vi "TCP Factory.vi"(8 "error in (no error)":errorcluster, 10 "TCP Settings":cluster{"IP Address":string, "Port":u16}) -> (0 "error out":errorcluster, 3 "TCP out":refnum<class "TCP.lvclass">)   [LabVIEW 2019, in "Protocols.lvlib" / "TCP.lvclass"]
uses:
  TCP.lvclass
  TCP.lvclass/TCP.ctl
  Data Access/Write IP Address.vi
  Data Access/Write Port.vi
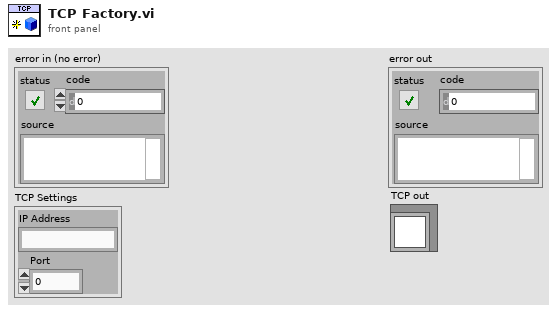
[diagram p1: front panel]
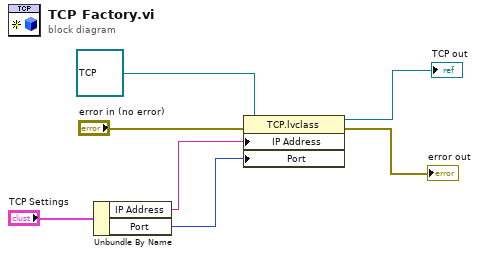
[diagram p0: block diagram]
diagram:
  n1 = Unbundle By Name("TCP Settings") -> ("IP Address"=w2:string, "Port"=w1:u16)
  n2 = property class="TCP.lvclass"(reference=refnum<class "TCP.lvclass"> refnum ("Protocols.lvlib:TCP.lvclass"), error in="error in (no error)", "IP Address"=w2, "Port"=w1) -> (reference out=→"TCP out":refnum<class "TCP.lvclass">, error out=→"error out":errorcluster)
